vi "IdentifySearchNode.vi"(8 "error in (no error)":errorcluster, 10 "NodeToIdentify in":refnum<data-value>, 11 "PriorityQueue in":refnum<class "PriorityQueue.lvclass">) -> (0 "error out":errorcluster, 1 "IsNode":bool, 2 "NodeToIdentify out":refnum<data-value>, 3 "PriorityQueue out":refnum<class "PriorityQueue.lvclass">)   [LabVIEW 2009, in "PriorityQueue.lvclass"]
uses:
  PriorityQueue.lvclass
  LLNode/LLNode.lvclass
  PriorityNode/PriorityNode.lvclass
  PriorityQueue.lvclass/PriorityQueue.ctl
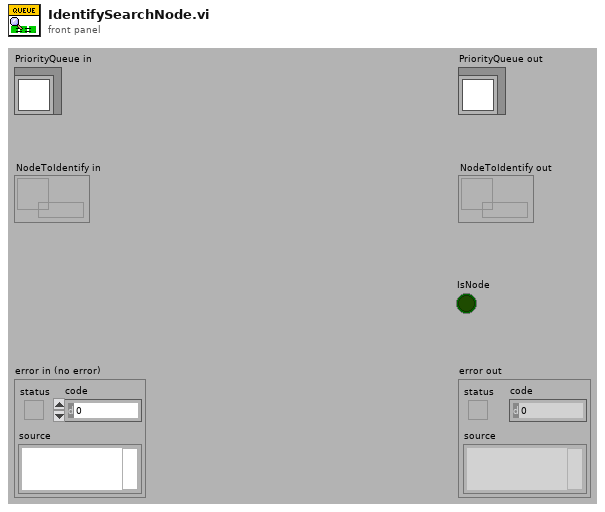
[diagram p1: front panel]
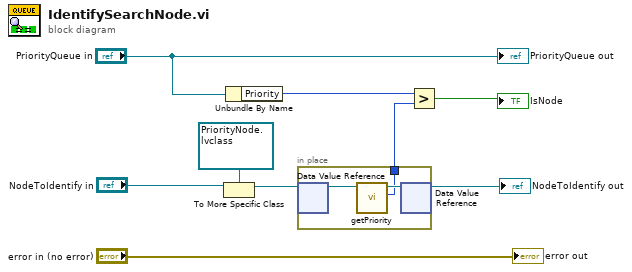
[diagram p0: block diagram]
diagram:
  n1 = To More Specific Class(target class=refnum<data-value> refnum ("data value reference"), reference="NodeToIdentify in") -> (specific class reference=w8:refnum<data-value>)  [unwired: 1 in, 1 out]
  n2 = Unbundle By Name("PriorityQueue in") -> ("Priority"=w6:u8)
  n3 = in-place {
    in-place-border: [w10] -> w7
    n4 = in-place-dvr #1(w8) -> (w12:refnum<class "PriorityNode.lvclass">)  [unwired: 1 out]
    n5 = call "getPriority.vi"("PriorityNode in"=w12) -> ("Priority"=w10:u8, "PriorityNode out"=w11:refnum<class "PriorityNode.lvclass">)  [unwired: 8 in, 1 out]
    n6 = in-place-dvr #1(w11) -> (→"NodeToIdentify out":refnum<data-value>)  [unwired: 1 out]
  }
  n7 = Greater?(x=w6, y=w7) -> (0:→"IsNode":bool)
  "error out" <- "error in (no error)"
  "PriorityQueue out" <- "PriorityQueue in"
